vi "WILT.vi"() -> ()   [LabVIEW 2016] (continued)
                n1233 = Not(x=w2304) -> (.not. x?=w2315:bool)
                n1234 = call "WILT Agilent Valve Control.vi"("Station In"=w2316, "Agilent Channels In"=w2312, "Semaphore"=w2314, "Search"=T19 "Start Button", "Open/Close (F:Close)"=w2315, "error in (no error)"=w2311, "Test Type"=w2307, "Number Of Cycles"=w2306, "Cycle Time (mS)"=w2305) -> ("error out"=w2310:errorcluster)  [unwired: 4 in, 2 out]
              }
            }
            n1235 = call <vilib>:"Add State(s) to Queue__jki_lib_state_machine.vi"("State(s) in (\"\")"=w2302) -> ("States Out"=w2301:string)  [unwired: 14 in]
          }
          event Value Change {
            n1236 = event-data() -> ("NewVal"=w2317:bool)  [unwired: 1 in, 1 out]
            n1237 = case shown="False" w2317 {
              tunnel: w2320 -> [_ w2333]
              tunnel: w2319 -> [w2323 w2331]
              tunnel: [w2323 w2330] -> w2318
              tunnel: w2317 -> [_ w2324]
              frame False {
              }
              frame True {
                n1238 = local read "Number of ON/OFF Cycles"() -> (w2326:i32)
                n1239 = local read "Valve ON Time (mS)"() -> (w2325:u32)
                n1240 = local read "Agilent Semaphore"() -> (w2334:T1[])
                n1241 = Unbundle By Name(w2333) -> ("Agilent Switches"=w2332:T2[])
                n1242 = local read "Test Type"() -> (w2327:T12)
                n1243 = Number To Decimal String(number=55) -> (decimal integer string=w2336:string)  [unwired: 1 in]
                n1244 = Not(x=w2324) -> (.not. x?=w2335:bool)
                n1245 = call "WILT Agilent Valve Control.vi"("Station In"=w2336, "Agilent Channels In"=w2332, "Semaphore"=w2334, "Search"=T19 "Start Button", "Open/Close (F:Close)"=w2335, "error in (no error)"=w2331, "Test Type"=w2327, "Number Of Cycles"=w2326, "Cycle Time (mS)"=w2325) -> ("error out"=w2330:errorcluster)  [unwired: 4 in, 2 out]
              }
            }
            n1246 = call <vilib>:"Add State(s) to Queue__jki_lib_state_machine.vi"("State(s) in (\"\")"=w2322) -> ("States Out"=w2321:string)  [unwired: 14 in]
          }
          event Value Change {
            n1247 = event-data() -> ("NewVal"=w2337:bool)  [unwired: 1 in, 1 out]
            n1248 = case shown="False" w2337 {
              tunnel: w2340 -> [_ w2353]
              tunnel: w2339 -> [w2343 w2351]
              tunnel: [w2343 w2350] -> w2338
              tunnel: w2337 -> [_ w2344]
              frame False {
              }
              frame True {
                n1249 = local read "Number of ON/OFF Cycles"() -> (w2346:i32)
                n1250 = local read "Valve ON Time (mS)"() -> (w2345:u32)
                n1251 = local read "Agilent Semaphore"() -> (w2354:T1[])
                n1252 = Unbundle By Name(w2353) -> ("Agilent Switches"=w2352:T2[])
                n1253 = local read "Test Type"() -> (w2347:T12)
                n1254 = Number To Decimal String(number=56) -> (decimal integer string=w2356:string)  [unwired: 1 in]
                n1255 = Not(x=w2344) -> (.not. x?=w2355:bool)
                n1256 = call "WILT Agilent Valve Control.vi"("Station In"=w2356, "Agilent Channels In"=w2352, "Semaphore"=w2354, "Search"=T19 "Start Button", "Open/Close (F:Close)"=w2355, "error in (no error)"=w2351, "Test Type"=w2347, "Number Of Cycles"=w2346, "Cycle Time (mS)"=w2345) -> ("error out"=w2350:errorcluster)  [unwired: 4 in, 2 out]
              }
            }
            n1257 = call <vilib>:"Add State(s) to Queue__jki_lib_state_machine.vi"("State(s) in (\"\")"=w2342) -> ("States Out"=w2341:string)  [unwired: 14 in]
          }
          event User Event {
            n1258 = event-data() -> ()  [unwired: 1 in, 3 out]
            n1259 = Unbundle By Name(w2362) -> ("GUI Aisle 1 (SLAT)."=w2359:T3[])
            n1260 = local read "Aisle 1 Update"() -> (w2357:T3)
            n1261 = local read "Aisle 1 Location"() -> (w2358:i32)
            n1262 = call "WILT Update Aisle Info.vi"("Aisle 4 Update"=w2357, "Aisle 4 Location"=w2358, "GUI Aisle 4. in"=w2359) -> ("GUI Aisle 4. out"=w2360:T3[])  [unwired: 8 in]
            n1263 = Bundle By Name(cluster=w2362, "GUI Aisle 1 (SLAT)."=w2360) -> (w2361:T24)
          }
          event User Event {
            n1264 = event-data() -> ()  [unwired: 1 in, 5 out]
            n1265 = Unbundle By Name(w2370) -> ("GUI Aisle 1A (SLAT)."=w2367:T3[])
            n1266 = local read "Aisle 1A Location"() -> (w2366:i32)
            n1267 = local read "Aisle 1A Update"() -> (w2365:T3)
            n1268 = call "WILT Update Aisle Info.vi"("Aisle 4 Update"=w2365, "Aisle 4 Location"=w2366, "GUI Aisle 4. in"=w2367) -> ("GUI Aisle 4. out"=w2368:T3[])  [unwired: 8 in]
            n1269 = Bundle By Name(cluster=w2370, "GUI Aisle 1A (SLAT)."=w2368) -> (w2369:T24)
          }
          event User Event {
            n1270 = event-data() -> ()  [unwired: 1 in, 5 out]
            n1271 = Unbundle By Name(w2378) -> ("GUI Aisle 2."=w2375:T3[])
            n1272 = local read "Aisle 2 Location"() -> (w2374:i32)
            n1273 = local read "Aisle 2 Update"() -> (w2373:T3)
            n1274 = call "WILT Update Aisle Info.vi"("Aisle 4 Update"=w2373, "Aisle 4 Location"=w2374, "GUI Aisle 4. in"=w2375) -> ("GUI Aisle 4. out"=w2376:T3[])  [unwired: 8 in]
            n1275 = Bundle By Name(cluster=w2378, "GUI Aisle 2."=w2376) -> (w2377:T24)
          }
          event User Event {
            n1276 = event-data() -> ()  [unwired: 1 in, 5 out]
            n1277 = Unbundle By Name(w2386) -> ("GUI Aisle 3."=w2383:T3[])
            n1278 = local read "Aisle 3 Location"() -> (w2382:i32)
            n1279 = local read "Aisle 3 Update"() -> (w2381:T3)
            n1280 = call "WILT Update Aisle Info.vi"("Aisle 4 Update"=w2381, "Aisle 4 Location"=w2382, "GUI Aisle 4. in"=w2383) -> ("GUI Aisle 4. out"=w2384:T3[])  [unwired: 8 in]
            n1281 = Bundle By Name(cluster=w2386, "GUI Aisle 3."=w2384) -> (w2385:T24)
          }
          event User Event {
            n1282 = event-data() -> ()  [unwired: 1 in, 5 out]
            n1283 = local read "Aisle 4 Location"() -> (w2389:i32)
            n1284 = local read "Aisle 4 Update"() -> (w2391:T3)
            n1285 = Unbundle By Name(w2394) -> ("GUI Aisle 4."=w2390:T3[])
            n1286 = call "WILT Update Aisle Info.vi"("Aisle 4 Update"=w2391, "Aisle 4 Location"=w2389, "GUI Aisle 4. in"=w2390) -> ("GUI Aisle 4. out"=w2392:T3[])  [unwired: 8 in]
            n1287 = Bundle By Name(cluster=w2394, "GUI Aisle 4."=w2392) -> (w2393:T24)
          }
          event Value Change {
            n1288 = event-data() -> ("NewVal"=w2398:T11)  [unwired: 1 in, 5 out]
            n1289 = case shown="\"Night Cycle\"" w2398 {
              tunnel: ["Reset Start Retry" ("State(s) in Front (\"\")") "Reset Start Retry\nShutdown All Valves" ("State(s) in Front (\"\")")] -> w2397
              frame "Day Cycle", Default {
              }
              frame "Night Cycle" {
              }
            }
            n1290 = call <vilib>:"Add State(s) to Queue__jki_lib_state_machine.vi"("State(s) in Front (\"\")"=w2397, "State(s) in (\"\")"=w2400) -> ("States Out"=w2399:string)  [unwired: 13 in]
          }
          event "Shutdown All Valves": Value Change {
            n1291 = event-data() -> ("NewVal"=w2406:bool)  [unwired: 1 in, 5 out]
            n1292 = case shown="True" w2406 {
              tunnel: ["" ("State(s) in Front (\"\")") "Shutdown All Valves" ("State(s) in Front (\"\")")] -> w2405
              frame False {
              }
              frame True {
                n1293 = local write "Shutdown All Valves"(FALSE ("Shutdown All Valves")) -> ()
              }
            }
            n1294 = call <vilib>:"Add State(s) to Queue__jki_lib_state_machine.vi"("State(s) in Front (\"\")"=w2405, "State(s) in (\"\")"=w2408) -> ("States Out"=w2407:string)  [unwired: 13 in]
          }
          event "Reset Start Retry": Value Change {
            n1295 = event-data() -> ("NewVal"=w2415:bool)  [unwired: 1 in, 5 out]
            n1296 = case shown="True" w2415 {
              tunnel: ["" ("State(s) in Front (\"\")") "Reset Start Retry" ("State(s) in Front (\"\")")] -> w2414
              frame False {
              }
              frame True {
                n1297 = local write "Reset Start Retry"(FALSE ("Reset Start Retry")) -> ()
              }
            }
            n1298 = call <vilib>:"Add State(s) to Queue__jki_lib_state_machine.vi"("State(s) in Front (\"\")"=w2414, "State(s) in (\"\")"=w2417) -> ("States Out"=w2418:string)  [unwired: 13 in]
          }
          event "Reset Start Retry All True": Value Change {
            n1299 = event-data() -> ("NewVal"=w2424:bool)  [unwired: 1 in, 5 out]
            n1300 = case shown="True" w2424 {
              tunnel: ["" ("State(s) in Front (\"\")") "Reset Restart All True" ("State(s) in Front (\"\")")] -> w2423
              frame False {
              }
              frame True {
                n1301 = local write "Reset Start Retry All True"(FALSE ("Reset Start Retry")) -> ()
              }
            }
            n1302 = call <vilib>:"Add State(s) to Queue__jki_lib_state_machine.vi"("State(s) in Front (\"\")"=w2423, "State(s) in (\"\")"=w2426) -> ("States Out"=w2427:string)  [unwired: 13 in]
          }
          event "ExitProg": Value Change {
            n1303 = event-data() -> ()  [unwired: 1 in, 1 out]
            n1304 = call <vilib>:"Add State(s) to Queue__jki_lib_state_machine.vi"("State(s) in Front (\"\")"="Shutdown All Valves\nMacro: Exit", "State(s) in (\"\")"=w2436) -> ("States Out"=w2435:string)  [unwired: 13 in]
          }
          event Panel Close? {
            # "Discard the event because we'll close the front panel ourselves in Macro: Exit"
            # "Close Panel button (pressed) Event\n(this executes Macro: Exit to terminate the VI)"
            n1305 = event-data() -> ()  [unwired: 1 in, 1 out]
            n1306 = event-data("Discard?"=TRUE) -> ()  [unwired: 1 in, 1 out]
            n1307 = call <vilib>:"Add State(s) to Queue__jki_lib_state_machine.vi"("State(s) in Front (\"\")"="Macro: Exit", "State(s) in (\"\")"=w2442) -> ("States Out"=w2441:string)  [unwired: 13 in]
          }
        }
      }
      frame "---------- Core ----------" {
        n1308 = call <vilib>:"Add State(s) to Queue__jki_lib_state_machine.vi"("State(s) in (\"\")"=w2447) -> ("States Out"=w2446:string)  [unwired: 14 in]
      }
      frame Default {
        w2458 = 42 items=["No error", "Argument error", "Memory is full", "Out of zone", "End of file", "File already open", "Generic file I/O error", "File not found", "File permission error", "Disk is full", "Duplicate path", "Too many files open", "System feature not enabled", "Resource file not found", "Cannot add resource", "Resource not found", "Image not found", "Image memory error", "Pen does not exist", "Config type invalid", "Config token not found", "Config parse error", "Config memory error", "Bad external code format", "Bad external code offset", "External code not present", "Null window", "Destroy window error", "Null menu", "Print aborted", "Bad print record", "Print driver error", "Windows error during printing", "Memory error during printing", "Print dialog error", "Generic print error", "Invalid device refnum", "Device not found", "Device parameter error", "Device unit error", "Cannot open device", "Device call aborted", "Generic error", "Cancelled by user", "Object ID too low", "Object ID too high", "Object not in heap", "Unknown heap", "Unknown object (invalid DefProc)", "Unknown object (DefProc not in table)", "Message out of range", "Invalid (null) method", "Unknown message", "Manager call not supported", "Bad address", "Network operation in progress", "Network operation timed out", "Connection is busy", "Network attribute not supported", "Network error", "Address in use", "System out of memory", "Connection aborted", "Connection refused", "Not connected", "Already connected", "Connection closed", "Initialization error (interapplication manager)", "Bad occurrence", "Wait on unbound occurrence handler", "Occurrence queue overflow", "Datalog type conflict", "Unused", "Unrecognized type (interapplication manager)", "Memory corrupt", "Failed to make temporary DLL", "Old CIN version", "Drag socket not found", "Failed to load drop-object", "Failed to register OLE object", "Failed to release OLE object", "Format specifier type mismatch", "Unknown format specifier", "Too few format specifiers", "Too many format specifiers", "Scan failed", "Newer CIN version", "Error converting to variant", "Runtime menu error", "Password tampered", "Variant attribute not found", "Incompatible variant data type", "Event data is not available", "Event Store is not present", "Occurrence is not found", "Event Queue is not created", "Event info is not available", "Refnum passed is NULL", "Error retrieving Class GUID", "Error retrieving CoClass GUID", "Error retrieving TypeLib GUID.", "Bad built application magic bytes.", "Specific driver is different from the specific driver associated with the Logical Name.", "There is no session opened to the class driver.", "Max Error", "MAX - Error with config objects", "MAX - Error loading configuration", "MAX - Group not supported"]
        # "Current State"
        # "Do not delete, rename, or modify this frame.\n(this is used to capture unhandled states and typos)"
        # "Handle mistyped state name (developer tool)"
        n1309 = Format Into String(format string="Software Exception: Unhandled State \"%s\"." ("message"), error in=w2454, w2449) -> (resulting string=w2457:string, error out=w2456:errorcluster)  [unwired: 1 in]
        n1310 = call <vilib>:"Error Cluster From Error Code.vi"("show call chain? (False)"=TRUE, "error in (no error)"=w2456, "error message (\"\")"=w2457, "error code (0)"=w2458) -> ("error out"=w2455:errorcluster)  [unwired: 5 in]
        n1311 = call <vilib>:"Add State(s) to Queue__jki_lib_state_machine.vi"("State(s) in (\"\")"=w2453) -> ("States Out"=w2452:string)  [unwired: 14 in]
      }
      frame "Initialize Core Data" {
        # "Do not delete, rename, or modify this frame.\n(this is used to determine panel behavior on exit)"
        # "originally closed?"
        # "exe?"
        # "If panel starts closed or is an EXE, then close it when we exit"
        n1312 = property class="VI"() -> ("Front Panel.Open"=w2468:bool)  [unwired: 2 in, 2 out]
        n1313 = property class="App"() -> ("App.Kind"=w2467:T20)  [unwired: 2 in, 2 out]
        n1314 = control-ref of="Current VI Reference"() -> (w2461:refnum<vi>)
        n1315 = Not(x=w2468) -> (.not. x?=w2465:bool)
        n1316 = Equal?(x=w2467, y=T20."Run Time System" ("Application:Kind")) -> (x = y?=w2464:bool)
        n1317 = Or(x=w2465, y=w2464) -> (x .or. y?=w2462:bool)
        n1318 = Bundle By Name(cluster=w2463, "Core.Current VI Reference"=w2461, "Core.Close Panel on Exit?"=w2462) -> (w2470:T24)
        n1319 = call <vilib>:"Add State(s) to Queue__jki_lib_state_machine.vi"("State(s) in (\"\")"=w2472) -> ("States Out"=w2471:string)  [unwired: 14 in]
      }
      frame "Error Handler" {
        # "Unhandled Error -- Display it"
        # "Handle any errors here.\nYou can also output any states to clean-up after errors occur"
        # "Clear error"
        n1320 = call <vilib>:"General Error Handler.vi"("error in (no error)"=w2475) -> ()  [unwired: 10 in, 5 out]
        n1321 = call <vilib>:"Add State(s) to Queue__jki_lib_state_machine.vi"("State(s) in Front (\"\")"="/* Post Error States", "State(s) in (\"\")"=w2479) -> ("States Out"=w2478:string)  [unwired: 13 in]
      }
      frame "Exit" {
        # "Do not put any code in this frame.\n(No errors that occur here will be handled.)"
        n1322 = call <vilib>:"Add State(s) to Queue__jki_lib_state_machine.vi"("State(s) in (\"\")"=w2485) -> ("States Out"=w2484:string)  [unwired: 14 in]
      }
      frame "---------- Data ----------" {
        # "Do not put any code in this frame.\n(It is a separator no-op. You can make a copy of this frame to create a new Data frame)"
        n1323 = call <vilib>:"Add State(s) to Queue__jki_lib_state_machine.vi"("State(s) in (\"\")"=w2490) -> ("States Out"=w2489:string)  [unwired: 14 in]
      }
      frame "Data: Initialize" {
        w2495 = 0.0  # Send Restart Every? (Sec)
        w2496 = bool[] [FALSE, FALSE, FALSE, FALSE, FALSE, FALSE, FALSE, FALSE, FALSE, FALSE, FALSE, FALSE, FALSE, FALSE, FALSE, FALSE, FALSE, FALSE, FALSE, FALSE, FALSE, FALSE, FALSE, FALSE, FALSE, FALSE, FALSE, FALSE, FALSE, FALSE, FALSE, FALSE, FALSE, FALSE, FALSE, FALSE, FALSE, FALSE, FALSE, FALSE, FALSE, FALSE, FALSE, FALSE, FALSE, FALSE, FALSE, FALSE, FALSE, FALSE, FALSE, FALSE, FALSE, FALSE, FALSE, FALSE]  # Enable Start Retry Array
        w2500 = 1.0  # Current Threshold
        w2512 = T25 {"Current VI Reference"=refnum, "Close Panel on Exit?"=FALSE}  # Core
        n1324 = Bundle("Send Restart Every? (Sec)"=w2495, "Enable Start Retry Array"=w2496, "Agilent Switches"="Agilent Switches", "States"="", "Core"=w2512, "Station Test State Cluster"="Station Test State Cluster", "GUI Aisle 4."="GUI Aisle 4.", "GUI Aisle 3."="GUI Aisle 3.", "GUI Aisle 2."="GUI Aisle 2.", "GUI Aisle 1A (SLAT)."="GUI Aisle 1A (SLAT).", "GUI Aisle 1 (SLAT)."="GUI Aisle 1 (SLAT).", "Agilent Refs"="Agilent Refs", "Configuration Startup Directorys"=T21 {"Debug File DIR"="", "Inverter And MC File DIR"=""}, "File Locations"="File Locations", "Day/Night Cycle Input"=WILT_Day_Night_Cycle_Enum."Day Cycle", "Injection Times Input"=T15 [], "Current Threshold"=w2500, "Station Timeout Values (1-56) Seconds"="Station Timeout Values (1-56) Seconds", "Drying Time (Min)"="Drying Time (Min)") -> (w2492:T24)  [unwired: 1 in]
        n1325 = call <vilib>:"Add State(s) to Queue__jki_lib_state_machine.vi"("State(s) in (\"\")"=w2514) -> ("States Out"=w2513:string)  [unwired: 14 in]
      }
      frame "Data: Cleanup" {
        # "Cleanup any data and references, here.\n(this is called automatically, by the Macro: Exit)"
        n1326 = Unbundle By Name(w2516) -> ("Core.Current VI Reference"=w2519:refnum<vi>)
        n1327 = Close Reference(reference=w2519, error in (no error)=w2518) -> (error out=w2517:errorcluster)
        n1328 = call <vilib>:"Add State(s) to Queue__jki_lib_state_machine.vi"("State(s) in (\"\")"=w2521) -> ("States Out"=w2520:string)  [unwired: 14 in]
      }
      frame "---------- UI ----------" {
        # "Do not put any code in this frame.\n(It is a separator no-op. You can make a copy of this frame to create a new UI frame)"
        n1329 = call <vilib>:"Add State(s) to Queue__jki_lib_state_machine.vi"("State(s) in (\"\")"=w2526) -> ("States Out"=w2525:string)  [unwired: 14 in]
      }
      frame "UI: Initialize" {
        # "Initialize everything so it starts without a serial number.\nThis prevents from running"
        n1330 = Current VI's Path() -> (path=w2531:path)
        n1331 = Unbundle By Name(w2533) -> ("File Locations"=w2532:T17[])
        n1332 = call "UTILITY This VIs Path.vi"("path"=w2531, "error in (no error)"=w2530) -> ("Folder Path"=w2528:path, "error out"=w2529:errorcluster)  [unwired: 7 in, 5 out]
        n1333 = for {
          tunnel: w2532 -> [w2547] mode=indexing
          tunnel: w2528 -> [w2546]
          tunnel: [w2545] -> w2527 mode=indexing
          n1334 = Bundle By Name(cluster=w2547, "General Setup Paths.Tool Base Path"=w2546) -> (w2545:T17)
        }
        n1335 = Initialize Array(T3 {"Lab ID"="", "Day Cycle Count"=0, "Station Label"="", "Dryer Details"={"Station"="", "Lab ID"="", "TR Number"=""}, "Status Color"=0, "Invisible Button"=FALSE, "Night Cycle Count"=0, "Station Index"=0, "Cycle Index"="", "Audit Alert"=FALSE, "Agilent Channel Definition"={"Channel"="", "Station"="", "Label"="", "Agilent Station"="", "Data"=0.0}, "DAQ Data"={"L1 Current"=0.0, "L2 Current"=0.0, "Temperature  Deg F (TC)"=0.0, "Volts"=0.0, "Volts (208)"=0.0, "SW (208)"=0.0}} ("Initial Dryer Cluster"), 12 ("dimension size")) -> (w2539:T3[])
        n1336 = Initialize Array(T3 {"Lab ID"="", "Day Cycle Count"=0, "Station Label"="", "Dryer Details"={"Station"="", "Lab ID"="", "TR Number"=""}, "Status Color"=0, "Invisible Button"=FALSE, "Night Cycle Count"=0, "Station Index"=0, "Cycle Index"="", "Audit Alert"=FALSE, "Agilent Channel Definition"={"Channel"="", "Station"="", "Label"="", "Agilent Station"="", "Data"=0.0}, "DAQ Data"={"L1 Current"=0.0, "L2 Current"=0.0, "Temperature  Deg F (TC)"=0.0, "Volts"=0.0, "Volts (208)"=0.0, "SW (208)"=0.0}} ("Initial Dryer Cluster"), 8 ("dimension size")) -> (w2536:T3[])
        n1337 = Bundle By Name(cluster=w2533, "Station Test State Cluster"=T7 {"Station Test State 1"=enum."No Serial Number", "Station Test State 2"=enum."No Serial Number", "Station Test State 3"=enum."No Serial Number", "Station Test State 4"=enum."No Serial Number", "Station Test State 5"=enum."No Serial Number", "Station Test State 6"=enum."No Serial Number", "Station Test State 7"=enum."No Serial Number", "Station Test State 8"=enum."No Serial Number", "Station Test State 9"=enum."No Serial Number", "Station Test State 10"=enum."No Serial Number", "Station Test State 11"=enum."No Serial Number", "Station Test State 12"=enum."No Serial Number", "Station Test State 13"=enum."No Serial Number", "Station Test State 14"=enum."No Serial Number", "Station Test State 15"=enum."No Serial Number", "Station Test State 16"=enum."No Serial Number", "Station Test State 17"=enum."No Serial Number", "Station Test State 18"=enum."No Serial Number", "Station Test State 19"=enum."No Serial Number", "Station Test State 20"=enum."No Serial Number", "Station Test State 21"=enum."No Serial Number", "Station Test State 22"=enum."No Serial Number", "Station Test State 23"=enum."No Serial Number", "Station Test State 24"=enum."No Serial Number", "Station Test State 25"=enum."No Serial Number", "Station Test State 26"=enum."No Serial Number", "Station Test State 27"=enum."No Serial Number", "Station Test State 28"=enum."No Serial Number", "Station Test State 29"=enum."No Serial Number", "Station Test State 30"=enum."No Serial Number", "Station Test State 31"=enum."No Serial Number", "Station Test State 32"=enum."No Serial Number", "Station Test State 33"=enum."No Serial Number", "Station Test State 34"=enum."No Serial Number", "Station Test State 35"=enum."No Serial Number", "Station Test State 36"=enum."No Serial Number", "Station Test State 37"=enum."No Serial Number", "Station Test State 38"=enum."No Serial Number", "Station Test State 39"=enum."No Serial Number", "Station Test State 40"=enum."No Serial Number", "Station Test State 41"=enum."No Serial Number", "Station Test State 42"=enum."No Serial Number", "Station Test State 43"=enum."No Serial Number", "Station Test State 44"=enum."No Serial Number", "Station Test State 45"=enum."No Serial Number", "Station Test State 46"=enum."No Serial Number", "Station Test State 47"=enum."No Serial Number", "Station Test State 48"=enum."No Serial Number", "Station Test State 49"=enum."No Serial Number", "Station Test State 50"=enum."No Serial Number", "Station Test State 51"=enum."No Serial Number", "Station Test State 52"=enum."No Serial Number", "Station Test State 53"=enum."No Serial Number", "Station Test State 54"=enum."No Serial Number", "Station Test State 55"=enum."No Serial Number", "Station Test State 56"=enum."No Serial Number"}, "GUI Aisle 4."=w2539, "GUI Aisle 3."=w2539, "GUI Aisle 2."=w2539, "GUI Aisle 1 (SLAT)."=w2539, "GUI Aisle 1A (SLAT)."=w2536, "File Locations"=w2527) -> (w2542:T24)
        n1338 = call <vilib>:"Add State(s) to Queue__jki_lib_state_machine.vi"("State(s) in (\"\")"=w2544) -> ("States Out"=w2543:string)  [unwired: 14 in]
      }
      frame "Read General Config" {
        # "Populate the general file path settings"
        n1339 = Unbundle By Name(w2555) -> ("File Locations"=w2550:T17[])
        n1340 = call "WILT Read General Configuration.vi"("File Path Input"=w2550, "Error In"=w2559) -> ("Scan Rate"=w2554:dbl, "Save Rate"=w2553:dbl, "Current Threshold"=w2552:dbl, "Send Restart Every? (Sec)"=w2551:dbl, "State Machine String"=w2557:string, "File Path Output"=w2549:T17[], "Station Timeout Values (1-56) Seconds"=w2556:dbl[], "Drying Time (Min)"=w2548:dbl[], "Error Out"=w2558:errorcluster)  [unwired: 9 in]
        n1341 = local write "Drying Time (Min)"(w2548) -> ()
        n1342 = Bundle By Name(cluster=w2555, "Send Restart Every? (Sec)"=w2551, "States"=w2557, "File Locations"=w2549, "Station Timeout Values (1-56) Seconds"=w2556, "Drying Time (Min)"=w2548) -> (w2561:T24)
        n1343 = local write "Scan Rate (Seconds)"(w2554) -> ()
        n1344 = local write "Save Rate (Seconds)"(w2553) -> ()
        n1345 = local write "Current Threshold"(w2552) -> ()
        n1346 = call <vilib>:"Add State(s) to Queue__jki_lib_state_machine.vi"("State(s) in (\"\")"=w2563) -> ("States Out"=w2562:string)  [unwired: 14 in]
      }
      frame "Read Previous" {
        n1347 = Unbundle By Name(w2571) -> ("File Locations"=w2564:T17[], "GUI Aisle 4."=w2566:T3[], "GUI Aisle 3."=w2567:T3[], "GUI Aisle 2."=w2568:T3[], "GUI Aisle 1 (SLAT)."=w2569:T3[], "GUI Aisle 1A (SLAT)."=w2570:T3[])
        n1348 = call "WILT Stave Status.vi"("GUI Aisle 4"=w2566, "Operation Type"=enum16{"Write", "Read"}."Read", "File Locations"=w2564, "GUI Aisle 3"=w2567, "GUI Aisle 2"=w2568, "GUI Aisle 1 (SLAT)"=w2569, "Error In"=w2578, "GUI Aisle 1A (SLAT)"=w2570) -> ("GUI Aisle 4 Out"=w2576:T3[], "GUI Aisle 3 Out"=w2575:T3[], "GUI Aisle 2 Out"=w2574:T3[], "GUI Aisle 1 (SLAT) Out"=w2573:T3[], "GUI Aisle 1A (SLAT) Out"=w2572:T3[], "Error Out"=w2577:errorcluster)  [unwired: 2 in]
        n1349 = local write "GUI Aisle 4."(w2576) -> ()
        n1350 = local write "GUI Aisle 3."(w2575) -> ()
        n1351 = local write "GUI Aisle 2."(w2574) -> ()
        n1352 = local write "GUI Aisle 1 (SLAT)."(w2573) -> ()
        n1353 = local write "GUI Aisle 1A (SLAT)."(w2572) -> ()
        n1354 = Bundle By Name(cluster=w2571, "GUI Aisle 4."=w2576, "GUI Aisle 3."=w2575, "GUI Aisle 2."=w2574, "GUI Aisle 1 (SLAT)."=w2573, "GUI Aisle 1A (SLAT)."=w2572) -> (w2580:T24)
        n1355 = call <vilib>:"Add State(s) to Queue__jki_lib_state_machine.vi"("State(s) in (\"\")"=w2582) -> ("States Out"=w2581:string)  [unwired: 14 in]
      }
      frame "Read Water Times" {
        n1356 = Unbundle By Name(w2586) -> ("File Locations"=w2587:T17[])
        n1357 = call "WILT Watering Times.vi"("Execution Type"=enum16{"Write", "Read"}."Read", "File Locations"=w2587) -> ("Watering Times Output"=w2585:T15)  [unwired: 8 in, 1 out]
        n1358 = local write "Injection Times"(w2585) -> ()
        n1359 = call <vilib>:"Add State(s) to Queue__jki_lib_state_machine.vi"("State(s) in (\"\")"=w2590) -> ("States Out"=w2589:string)  [unwired: 14 in]
      }
      frame "UI: Cursor Set" {
        # "Argument"
        n1360 = case shown="\"Idle\", Default" w2592 {
          tunnel: w2594 -> [w2599 w2601]
          tunnel: [w2598 w2600] -> w2593
          frame "Idle", Default {
            n1361 = call <vilib>:"Unset Busy.vi"("error in (no error)"=w2599) -> ("error out"=w2598:errorcluster)  [unwired: 10 in]
          }
          frame "Busy" {
            n1362 = call <vilib>:"Set Busy.vi"("error in (no error)"=w2601) -> ("error out"=w2600:errorcluster)  [unwired: 9 in, 1 out]
          }
        }
        n1363 = call <vilib>:"Add State(s) to Queue__jki_lib_state_machine.vi"("State(s) in (\"\")"=w2597) -> ("States Out"=w2596:string)  [unwired: 14 in]
      }
      frame "UI: Front Panel State" {
        # "Argument"
        # "Set Front Panel Open or Closed\n(Usage: \"UI: Front Panel State >> Open|Close\")"
        n1364 = Unbundle By Name(w2605) -> ("Core.Current VI Reference"=w2604:refnum<vi>)
        n1365 = case shown="\"Open\", Default" w2603 {
          tunnel: w2607 -> [w2613 w2626]
          tunnel: [w2615 w2627] -> w2606
          tunnel: w2604 -> [w2614 w2624]
          frame "Open", Default {
            n1366 = property class="VI"(reference=w2614, error in=w2613) -> (reference out=w2611:refnum<vi>, error out=w2612:errorcluster, "Front Panel.Open"=w2610:bool)
            n1367 = case shown="False" w2610 {
              tunnel: [w2618 w2621] -> w2615
              tunnel: w2612 -> [w2617 w2621]
              tunnel: w2611 -> [w2616 _]
              frame False {
                n1368 = invoke class="VI" method="FP.Open"(reference=w2616, error in=w2617, "Activate"=TRUE, "State"=T22."Standard") -> (error out=w2618:errorcluster)  [unwired: 1 in, 4 out]
              }
              frame True {
              }
            }
          }
          frame "Close" {
            n1369 = property class="VI"(reference=w2624, error in=w2626) -> (reference out=w2623:refnum<vi>, error out=w2625:errorcluster, "Front Panel.Open"=w2622:bool)
            n1370 = case shown="True" w2622 {
              tunnel: [w2628 w2631] -> w2627
              tunnel: w2625 -> [w2628 w2630]
              tunnel: w2623 -> [_ w2629]
              frame False {
              }
              frame True {
                n1371 = invoke class="VI" method="FP.Close"(reference=w2629, error in=w2630) -> (error out=w2631:errorcluster)  [unwired: 1 in, 2 out]
              }
            }
          }
        }
        n1372 = call <vilib>:"Add State(s) to Queue__jki_lib_state_machine.vi"("State(s) in (\"\")"=w2609) -> ("States Out"=w2608:string)  [unwired: 14 in]
      }
      frame "Initialize Agilents" {
        n1373 = local read "Agilent Semaphore"() -> (w2634:T1[])
        n1374 = Unbundle By Name(w2637) -> ("File Locations"=w2633:T17[], "Agilent Refs"=w2642:refnum<visa-resource-name>[])
        n1375 = call "WILT Agilent Setup.vi"("Custom Agilent List"=FALSE, "Agilent Semaphore"=w2634, "error in (no error)"=w2641, "Agilent Refs"=w2642, "File Locations"=w2633) -> ("error out"=w2640:errorcluster, "Data Out Array"=→"Data Out Array":T6, "Agilent Switches"=w2635:T2[])  [unwired: 4 in]
        n1376 = Bundle By Name(cluster=w2637, "Agilent Switches"=w2635) -> (w2636:T24)
        n1377 = call <vilib>:"Add State(s) to Queue__jki_lib_state_machine.vi"("State(s) in (\"\")"=w2644) -> ("States Out"=w2643:string)  [unwired: 14 in]
      }
      frame "Initialize File Names" {
        # "Dont create folders if Lab ID is blank"
        n1378 = Unbundle By Name(w2645) -> ("File Locations"=w2646:T17[], "GUI Aisle 1 (SLAT)."=w2658:T3[], "GUI Aisle 1A (SLAT)."=w2657:T3[], "GUI Aisle 2."=w2656:T3[], "GUI Aisle 3."=w2655:T3[], "GUI Aisle 4."=w2654:T3[])
        n1379 = Build Array (concatenate)(w2658, w2657, w2656, w2655, w2654) -> (w2653:T3[])
        n1380 = for {
          tunnel: w2653 -> [w2668] mode=indexing
          tunnel: [w2667] -> w2651 mode=indexing
          tunnel: w2646 -> [w2662] mode=indexing
          n1381 = call "WILT Dryer To Washer Control Converter File Save.vi"("Dryer 14"=w2668) -> ("Initialize.Washer In"=w2663:T26)  [unwired: 9 in, 1 out]
          n1382 = Unbundle By Name(w2663) -> ("Appliance Details.Appliance Common.Lab ID:"=w2664:string)
          n1383 = Equal?(x=w2664, y="") -> (x = y?=w2665:bool)
          n1384 = case shown="False" w2665 {
            tunnel: w2662 -> [w2672 w2673]
            tunnel: w2663 -> [w2671 _]
            tunnel: [w2670 w2673] -> w2667
            frame False {
              n1385 = call "Save File Create Filename and Directories.vi"("LV Program"=Save_File_DOE_LabView_Program."Dryer WILT", "Initialize.Washer In"=w2671, "File Paths In"=w2672) -> ("File Paths Out"=w2670:T17)  [unwired: 6 in, 2 out]
            }
            frame True {
            }
          }
        }
        n1386 = Initialize Array(refnum<file> refnum ("File Refnum"), 57 ("dimension size")) -> (→"File Refnums":refnum<file>[])
        n1387 = call <vilib>:"Add State(s) to Queue__jki_lib_state_machine.vi"("State(s) in (\"\")"=w2661) -> ("States Out"=w2660:string)  [unwired: 14 in]
        n1388 = Bundle By Name(cluster=w2645, "File Locations"=w2651) -> (w2652:T24)
        n1389 = local write "File Locations"(w2651) -> ()
      }
      frame "Shutdown All Valves" {
        n1390 = Unbundle By Name(w2683) -> ("Agilent Switches"=w2682:T2[])
        n1391 = global read "WILT Globals Main Program.vi" "Startup"() -> (→"Unused":u32)
        n1392 = global read "WILT Globals Main Program.vi" "Run"() -> (→"Running":u32)
        n1393 = global read "WILT Globals Main Program.vi" "Color Uncofigured"() -> (→"No Com":u32)
        n1394 = global read "WILT Globals Main Program.vi" "Problem"() -> (→"Fault":u32)
        n1395 = global read "WILT Globals Main Program.vi" "Pause"() -> (→"Stopped":u32)
        n1396 = global read "WILT Globals Main Program.vi" "Watering"() -> (→"Watering":u32)
        n1397 = global read "WILT Globals Main Program.vi" "EOC"() -> (→"Waiting For Start":u32)
        n1398 = local read "Agilent Semaphore"() -> (w2674:T1[])
        n1399 = call "WILT Shutdown All Valves.vi"("Agilent Semaphore"=w2674, "error in (no error)"=w2685, "Agilent Switches"=w2682) -> ("error out"=w2684:errorcluster)  [unwired: 8 in]
        n1400 = call <vilib>:"Add State(s) to Queue__jki_lib_state_machine.vi"("State(s) in (\"\")"=w2688) -> ("States Out"=w2687:string)  [unwired: 14 in]
      }
      frame "Initialization Complete" {
        n1401 = Current VI's Path() -> (path=w2695:path)
        n1402 = call "UTILITY This VIs Path.vi"("path"=w2695, "error in (no error)"=w2690) -> ("Robocopy Path"=w2691:string, "FileVersionInfo Out"=w2694:T28, "error out"=w2689:errorcluster)  [unwired: 7 in, 4 out]
        n1403 = Unbundle By Name(w2694) -> ("FileVersion"=→"Version":string)
        n1404 = call <vilib>:"System Exec.vi"("wait until completion? (T)"=FALSE, "command line"=w2691) -> ()  [unwired: 6 in, 4 out]
        n1405 = call <vilib>:"Add State(s) to Queue__jki_lib_state_machine.vi"("State(s) in (\"\")"=w2700) -> ("States Out"=w2699:string)  [unwired: 14 in]
        "Initialization Complete" <- TRUE ("Initialization Complete")
      }
      frame "Reset Start Retry" {
        n1406 = Initialize Array(FALSE, 56 ("dimension size")) -> (w2701:bool[])
        n1407 = Bundle By Name(cluster=w2705, "Enable Start Retry Array"=w2701) -> (w2704:T24)
        n1408 = call <vilib>:"Add State(s) to Queue__jki_lib_state_machine.vi"("State(s) in (\"\")"=w2709) -> ("States Out"=w2708:string)  [unwired: 14 in]
      }
      frame "Reset Restart All True" {
        n1409 = Initialize Array(TRUE, 56 ("dimension size")) -> (w2710:bool[])
        n1410 = Bundle By Name(cluster=w2714, "Enable Start Retry Array"=w2710) -> (w2713:T24)
        n1411 = call <vilib>:"Add State(s) to Queue__jki_lib_state_machine.vi"("State(s) in (\"\")"=w2718) -> ("States Out"=w2717:string)  [unwired: 14 in]
      }
      frame "Wait Seconds" {
        n1412 = call "UTILITY Delay mS.vi"("Error In"=w2721, "milliseconds to wait"=u32 20000) -> ("Error Out"=w2720:errorcluster)  [unwired: 13 in]
        n1413 = call <vilib>:"Add State(s) to Queue__jki_lib_state_machine.vi"("State(s) in (\"\")"=w2725) -> ("States Out"=w2724:string)  [unwired: 14 in]
      }
      frame "---------- Macro ----------" {
        # "Do not put any code in this frame.\n(It is a separator no-op. You can make a copy of this frame to create a new Macro frame)"
        n1414 = call <vilib>:"Add State(s) to Queue__jki_lib_state_machine.vi"("State(s) in (\"\")"=w2730) -> ("States Out"=w2729:string)  [unwired: 14 in]
      }
      frame "Macro: Initialize" {
        w2732 = "Data: Initialize\nInitialize Core Data\nUI: Initialize\nRead General Config\nRead Previous\nRead Water Times\nInitialize Agilents\nInitialize File Names\nShutdown All Valves\nInitialization Complete\nUI: Front Panel State >> Open"  # Data: Initialize Initialize Core Data UI: Initialize Read General Config Read Previous Read Water Times Initialize Agilents Initialize File Names Shutdown All Valves Initialization Complete UI: Front Panel State >> Open
        n1415 = call <vilib>:"Add State(s) to Queue__jki_lib_state_machine.vi"("State(s) in Front (\"\")"=w2732, "State(s) in (\"\")"=w2736) -> ("States Out"=w2735:string)  [unwired: 13 in]
      }
      frame "Macro: Exit" {
        # "Exit Macro\n(This is called once, when the VI exits)"
        n1416 = Unbundle By Name(w2744) -> ("Core.Close Panel on Exit?"=w2743:bool)
        n1417 = Select(t="UI: Front Panel State >> Close", s=w2743, f="") -> (s? t:f=w2740:string)
        n1418 = call <vilib>:"Add State(s) to Queue__jki_lib_state_machine.vi"("State(s) in (\"\")"=w2740, "State(s) at Back (\"\")"="Data: Cleanup\nExit") -> ("States Out"=w2738:string)  [unwired: 13 in]
        n1419 = call <vilib>:"Add State(s) to Queue__jki_lib_state_machine.vi"("State(s) in Front (\"\")"=w2738, "State(s) in (\"\")"=w2747) -> ("States Out"=w2746:string)  [unwired: 13 in]
      }
      frame "---------- New Category ----------" {
        # "Template Separator\n(You can make a copy of, or modify, this frame)"
        n1420 = call <vilib>:"Add State(s) to Queue__jki_lib_state_machine.vi"("State(s) in (\"\")"=w2752) -> ("States Out"=w2751:string)  [unwired: 14 in]
      }
      frame "Read Constants" {
        n1421 = Bundle By Name(cluster=w2757, "Day/Night Cycle Input"="Day/Night Cycle", "Injection Times Input"="Injection Times", "Current Threshold"="Current Threshold") -> (w2756:T24)
        n1422 = call <vilib>:"Add State(s) to Queue__jki_lib_state_machine.vi"("State(s) in (\"\")"=w2761) -> ("States Out"=w2760:string)  [unwired: 14 in]
      }
      frame "Station 1" {
        w2779 = 0  # Aisle Location Index
        w2782 = u32 1  # Station Number
        # "Clean this up with a control"
        # "Control the state of station 1"
        n1423 = Unbundle By Name(w2786) -> ("Enable Start Retry Array"=w2771:bool[], "Agilent Switches"=w2772:T2[], "GUI Aisle 1 (SLAT)."=w2784:T3[], "Drying Time (Min)"=w2766:dbl[], "Current Threshold"=w2773:dbl, "Station Test State Cluster"=w2777:T7, "Station Timeout Values (1-56) Seconds"=w2767:dbl[], "Send Restart Every? (Sec)"=w2769:dbl, "Injection Times Input"=w2774:T15, "Day/Night Cycle Input"=w2775:T11)
        n1424 = local read "Previous Run Statistics"() -> (w2768:T9[])
        n1425 = local read "Agilent Semaphore"() -> (w2765:T1[])
        n1426 = call "WILT Station Controller.vi"("Station Number"=w2782, "GUI Aisle in"=w2784, "Drying Time (Min)"=w2766, "Current Threshold"=w2773, "Station Test State In"=w2777, "Error In"=w2781, "Aisle Location Index"=w2779, "Cool Down Period (seconds)"=w2767, "Disable Flood Check"="Disable Flood Check", "Delay After Cutout (sec)"="Delay After Cutout (Sec)", "Previous Run Statistics"=w2768, "Send Restart Every? (Sec)"=w2769, "Agilent Valve and Switch Locations"=w2772, "Injection Times"=w2774, "Enable Start Retry"=w2771, "Day/Night Cycle"=w2775, "Final Start Presses"="Final Start Presses", "Semaphore"=w2765) -> ("GUI Aisle 1"=w2783:T3[], "Test Station Out"=w2778:T7, "Enable Start Retry Out"=w2770:bool[], "Error Out"=w2780:errorcluster)  [unwired: 5 in, 1 out]
        n1427 = Bundle By Name(cluster=w2786, "GUI Aisle 1 (SLAT)."=w2783, "Station Test State Cluster"=w2778, "Enable Start Retry Array"=w2770) -> (w2785:T24)
        n1428 = call <vilib>:"Add State(s) to Queue__jki_lib_state_machine.vi"("State(s) in (\"\")"=w2788) -> ("States Out"=w2787:string)  [unwired: 14 in]
      }
      frame "Station 2" {
        w2806 = 1  # Aisle Location Index
        w2809 = u32 2  # Station Number
        # "Control the state of station 2"
        n1429 = Unbundle By Name(w2813) -> ("Enable Start Retry Array"=w2797:bool[], "Agilent Switches"=w2799:T2[], "GUI Aisle 1 (SLAT)."=w2811:T3[], "Drying Time (Min)"=w2794:dbl[], "Current Threshold"=w2800:dbl, "Station Test State Cluster"=w2804:T7, "Station Timeout Values (1-56) Seconds"=w2795:dbl[], "Send Restart Every? (Sec)"=w2796:dbl, "Injection Times Input"=w2801:T15, "Day/Night Cycle Input"=w2802:T11)
        n1430 = local read "Disable Flood Check"() -> (w2789:bool)
        n1431 = local read "Delay After Cutout (Sec)"() -> (w2791:dbl)
        n1432 = local read "Final Start Presses"() -> (w2790:i32)
        n1433 = local read "Agilent Semaphore"() -> (w2792:T1[])
        n1434 = local read "Previous Run Statistics"() -> (w2793:T9[])
        n1435 = call "WILT Station Controller.vi"("Station Number"=w2809, "GUI Aisle in"=w2811, "Drying Time (Min)"=w2794, "Current Threshold"=w2800, "Station Test State In"=w2804, "Error In"=w2808, "Aisle Location Index"=w2806, "Cool Down Period (seconds)"=w2795, "Disable Flood Check"=w2789, "Delay After Cutout (sec)"=w2791, "Previous Run Statistics"=w2793, "Send Restart Every? (Sec)"=w2796, "Agilent Valve and Switch Locations"=w2799, "Injection Times"=w2801, "Enable Start Retry"=w2797, "Day/Night Cycle"=w2802, "Final Start Presses"=w2790, "Semaphore"=w2792) -> ("GUI Aisle 1"=w2810:T3[], "Test Station Out"=w2805:T7, "Enable Start Retry Out"=w2798:bool[], "Error Out"=w2807:errorcluster)  [unwired: 5 in, 1 out]
        n1436 = Bundle By Name(cluster=w2813, "GUI Aisle 1 (SLAT)."=w2810, "Station Test State Cluster"=w2805, "Enable Start Retry Array"=w2798) -> (w2812:T24)
        n1437 = call <vilib>:"Add State(s) to Queue__jki_lib_state_machine.vi"("State(s) in (\"\")"=w2815) -> ("States Out"=w2814:string)  [unwired: 14 in]
      }
      frame "Station 3" {
        w2833 = 2  # Aisle Location Index
        w2836 = u32 3  # Station Number
        # "Control the state of station 3"
        n1438 = Unbundle By Name(w2840) -> ("Enable Start Retry Array"=w2824:bool[], "Agilent Switches"=w2826:T2[], "GUI Aisle 1 (SLAT)."=w2838:T3[], "Drying Time (Min)"=w2820:dbl[], "Current Threshold"=w2827:dbl, "Station Test State Cluster"=w2831:T7, "Station Timeout Values (1-56) Seconds"=w2822:dbl[], "Send Restart Every? (Sec)"=w2823:dbl, "Injection Times Input"=w2828:T15, "Day/Night Cycle Input"=w2829:T11)
        n1439 = local read "Previous Run Statistics"() -> (w2821:T9[])
        n1440 = local read "Disable Flood Check"() -> (w2816:bool)
        n1441 = local read "Delay After Cutout (Sec)"() -> (w2818:dbl)
        n1442 = local read "Final Start Presses"() -> (w2817:i32)
        n1443 = local read "Agilent Semaphore"() -> (w2819:T1[])
        n1444 = call "WILT Station Controller.vi"("Station Number"=w2836, "GUI Aisle in"=w2838, "Drying Time (Min)"=w2820, "Current Threshold"=w2827, "Station Test State In"=w2831, "Error In"=w2835, "Aisle Location Index"=w2833, "Cool Down Period (seconds)"=w2822, "Disable Flood Check"=w2816, "Delay After Cutout (sec)"=w2818, "Previous Run Statistics"=w2821, "Send Restart Every? (Sec)"=w2823, "Agilent Valve and Switch Locations"=w2826, "Injection Times"=w2828, "Enable Start Retry"=w2824, "Day/Night Cycle"=w2829, "Final Start Presses"=w2817, "Semaphore"=w2819) -> ("GUI Aisle 1"=w2837:T3[], "Test Station Out"=w2832:T7, "Enable Start Retry Out"=w2825:bool[], "Error Out"=w2834:errorcluster)  [unwired: 5 in, 1 out]
        n1445 = call <vilib>:"Add State(s) to Queue__jki_lib_state_machine.vi"("State(s) in (\"\")"=w2842) -> ("States Out"=w2841:string)  [unwired: 14 in]
        n1446 = Bundle By Name(cluster=w2840, "GUI Aisle 1 (SLAT)."=w2837, "Station Test State Cluster"=w2832, "Enable Start Retry Array"=w2825) -> (w2839:T24)
      }
      frame "Station 4" {
        w2860 = 3  # Aisle Location Index
        w2863 = u32 4  # Station Number
        # "Control the state of station 4"
        n1447 = Unbundle By Name(w2867) -> ("Enable Start Retry Array"=w2852:bool[], "Agilent Switches"=w2853:T2[], "GUI Aisle 1 (SLAT)."=w2865:T3[], "Drying Time (Min)"=w2848:dbl[], "Current Threshold"=w2854:dbl, "Station Test State Cluster"=w2858:T7, "Station Timeout Values (1-56) Seconds"=w2849:dbl[], "Send Restart Every? (Sec)"=w2850:dbl, "Injection Times Input"=w2855:T15, "Day/Night Cycle Input"=w2856:T11)
        n1448 = local read "Delay After Cutout (Sec)"() -> (w2845:dbl)
        n1449 = local read "Final Start Presses"() -> (w2844:i32)
        n1450 = local read "Agilent Semaphore"() -> (w2846:T1[])
        n1451 = local read "Previous Run Statistics"() -> (w2847:T9[])
        n1452 = local read "Disable Flood Check"() -> (w2843:bool)
        n1453 = call "WILT Station Controller.vi"("Station Number"=w2863, "GUI Aisle in"=w2865, "Drying Time (Min)"=w2848, "Current Threshold"=w2854, "Station Test State In"=w2858, "Error In"=w2862, "Aisle Location Index"=w2860, "Cool Down Period (seconds)"=w2849, "Disable Flood Check"=w2843, "Delay After Cutout (sec)"=w2845, "Previous Run Statistics"=w2847, "Send Restart Every? (Sec)"=w2850, "Agilent Valve and Switch Locations"=w2853, "Injection Times"=w2855, "Enable Start Retry"=w2852, "Day/Night Cycle"=w2856, "Final Start Presses"=w2844, "Semaphore"=w2846) -> ("GUI Aisle 1"=w2864:T3[], "Test Station Out"=w2859:T7, "Enable Start Retry Out"=w2851:bool[], "Error Out"=w2861:errorcluster)  [unwired: 5 in, 1 out]
        n1454 = Bundle By Name(cluster=w2867, "GUI Aisle 1 (SLAT)."=w2864, "Station Test State Cluster"=w2859, "Enable Start Retry Array"=w2851) -> (w2866:T24)
        n1455 = call <vilib>:"Add State(s) to Queue__jki_lib_state_machine.vi"("State(s) in (\"\")"=w2869) -> ("States Out"=w2868:string)  [unwired: 14 in]
      }
      frame "Station 5" {
        w2887 = 4  # Aisle Location Index
        w2890 = u32 5  # Station Number
        # "Control the state of station 5"
        n1456 = Unbundle By Name(w2894) -> ("Enable Start Retry Array"=w2879:bool[], "Agilent Switches"=w2881:T2[], "GUI Aisle 1 (SLAT)."=w2892:T3[], "Drying Time (Min)"=w2875:dbl[], "Current Threshold"=w2880:dbl, "Station Test State Cluster"=w2885:T7, "Station Timeout Values (1-56) Seconds"=w2876:dbl[], "Send Restart Every? (Sec)"=w2877:dbl, "Injection Times Input"=w2882:T15, "Day/Night Cycle Input"=w2883:T11)
        n1457 = local read "Delay After Cutout (Sec)"() -> (w2872:dbl)
        n1458 = local read "Final Start Presses"() -> (w2871:i32)
        n1459 = local read "Agilent Semaphore"() -> (w2873:T1[])
        n1460 = local read "Previous Run Statistics"() -> (w2874:T9[])
        n1461 = local read "Disable Flood Check"() -> (w2870:bool)
        n1462 = call "WILT Station Controller.vi"("Station Number"=w2890, "GUI Aisle in"=w2892, "Drying Time (Min)"=w2875, "Current Threshold"=w2880, "Station Test State In"=w2885, "Error In"=w2889, "Aisle Location Index"=w2887, "Cool Down Period (seconds)"=w2876, "Disable Flood Check"=w2870, "Delay After Cutout (sec)"=w2872, "Previous Run Statistics"=w2874, "Send Restart Every? (Sec)"=w2877, "Agilent Valve and Switch Locations"=w2881, "Injection Times"=w2882, "Enable Start Retry"=w2879, "Day/Night Cycle"=w2883, "Final Start Presses"=w2871, "Semaphore"=w2873) -> ("GUI Aisle 1"=w2891:T3[], "Test Station Out"=w2886:T7, "Enable Start Retry Out"=w2878:bool[], "Error Out"=w2888:errorcluster)  [unwired: 5 in, 1 out]
        n1463 = call <vilib>:"Add State(s) to Queue__jki_lib_state_machine.vi"("State(s) in (\"\")"=w2896) -> ("States Out"=w2895:string)  [unwired: 14 in]
        n1464 = Bundle By Name(cluster=w2894, "GUI Aisle 1 (SLAT)."=w2891, "Station Test State Cluster"=w2886, "Enable Start Retry Array"=w2878) -> (w2893:T24)
      }
      frame "Station 6" {
        w2914 = 5  # Aisle Location Index
        w2917 = u32 6  # Station Number
        # "Control the state of station 6"
        n1465 = Unbundle By Name(w2921) -> ("Enable Start Retry Array"=w2906:bool[], "Agilent Switches"=w2908:T2[], "GUI Aisle 1 (SLAT)."=w2919:T3[], "Drying Time (Min)"=w2902:dbl[], "Current Threshold"=w2907:dbl, "Station Test State Cluster"=w2912:T7, "Station Timeout Values (1-56) Seconds"=w2903:dbl[], "Send Restart Every? (Sec)"=w2904:dbl, "Injection Times Input"=w2909:T15, "Day/Night Cycle Input"=w2910:T11)
        n1466 = local read "Delay After Cutout (Sec)"() -> (w2899:dbl)
        n1467 = local read "Final Start Presses"() -> (w2898:i32)
        n1468 = local read "Agilent Semaphore"() -> (w2900:T1[])
        n1469 = local read "Previous Run Statistics"() -> (w2901:T9[])
        n1470 = local read "Disable Flood Check"() -> (w2897:bool)
        n1471 = call "WILT Station Controller.vi"("Station Number"=w2917, "GUI Aisle in"=w2919, "Drying Time (Min)"=w2902, "Current Threshold"=w2907, "Station Test State In"=w2912, "Error In"=w2916, "Aisle Location Index"=w2914, "Cool Down Period (seconds)"=w2903, "Disable Flood Check"=w2897, "Delay After Cutout (sec)"=w2899, "Previous Run Statistics"=w2901, "Send Restart Every? (Sec)"=w2904, "Agilent Valve and Switch Locations"=w2908, "Injection Times"=w2909, "Enable Start Retry"=w2906, "Day/Night Cycle"=w2910, "Final Start Presses"=w2898, "Semaphore"=w2900) -> ("GUI Aisle 1"=w2918:T3[], "Test Station Out"=w2913:T7, "Enable Start Retry Out"=w2905:bool[], "Error Out"=w2915:errorcluster)  [unwired: 5 in, 1 out]
        n1472 = Bundle By Name(cluster=w2921, "GUI Aisle 1 (SLAT)."=w2918, "Station Test State Cluster"=w2913, "Enable Start Retry Array"=w2905) -> (w2920:T24)
        n1473 = call <vilib>:"Add State(s) to Queue__jki_lib_state_machine.vi"("State(s) in (\"\")"=w2923) -> ("States Out"=w2922:string)  [unwired: 14 in]
      }
      frame "Station 7" {
        w2941 = 6  # Aisle Location Index
        w2944 = u32 7  # Station Number
        # "Control the state of station 7"
        n1474 = Unbundle By Name(w2948) -> ("Enable Start Retry Array"=w2932:bool[], "Agilent Switches"=w2935:T2[], "GUI Aisle 1 (SLAT)."=w2946:T3[], "Drying Time (Min)"=w2929:dbl[], "Current Threshold"=w2934:dbl, "Station Test State Cluster"=w2939:T7, "Station Timeout Values (1-56) Seconds"=w2930:dbl[], "Send Restart Every? (Sec)"=w2931:dbl, "Injection Times Input"=w2936:T15, "Day/Night Cycle Input"=w2937:T11)
        n1475 = local read "Delay After Cutout (Sec)"() -> (w2926:dbl)
        n1476 = local read "Final Start Presses"() -> (w2925:i32)
        n1477 = local read "Agilent Semaphore"() -> (w2927:T1[])
        n1478 = local read "Previous Run Statistics"() -> (w2928:T9[])
        n1479 = local read "Disable Flood Check"() -> (w2924:bool)
        n1480 = call "WILT Station Controller.vi"("Station Number"=w2944, "GUI Aisle in"=w2946, "Drying Time (Min)"=w2929, "Current Threshold"=w2934, "Station Test State In"=w2939, "Error In"=w2943, "Aisle Location Index"=w2941, "Cool Down Period (seconds)"=w2930, "Disable Flood Check"=w2924, "Delay After Cutout (sec)"=w2926, "Previous Run Statistics"=w2928, "Send Restart Every? (Sec)"=w2931, "Agilent Valve and Switch Locations"=w2935, "Injection Times"=w2936, "Enable Start Retry"=w2932, "Day/Night Cycle"=w2937, "Final Start Presses"=w2925, "Semaphore"=w2927) -> ("GUI Aisle 1"=w2945:T3[], "Test Station Out"=w2940:T7, "Enable Start Retry Out"=w2933:bool[], "Error Out"=w2942:errorcluster)  [unwired: 5 in, 1 out]
        n1481 = Bundle By Name(cluster=w2948, "GUI Aisle 1 (SLAT)."=w2945, "Station Test State Cluster"=w2940, "Enable Start Retry Array"=w2933) -> (w2947:T24)
        n1482 = call <vilib>:"Add State(s) to Queue__jki_lib_state_machine.vi"("State(s) in (\"\")"=w2950) -> ("States Out"=w2949:string)  [unwired: 14 in]
      }
      frame "Station 8" {
        w2968 = 7  # Aisle Location Index
        w2971 = u32 8  # Station Number
        # "Control the state of station 8"
        n1483 = Unbundle By Name(w2975) -> ("Enable Start Retry Array"=w2959:bool[], "Agilent Switches"=w2962:T2[], "GUI Aisle 1 (SLAT)."=w2973:T3[], "Drying Time (Min)"=w2956:dbl[], "Current Threshold"=w2961:dbl, "Station Test State Cluster"=w2966:T7, "Station Timeout Values (1-56) Seconds"=w2957:dbl[], "Send Restart Every? (Sec)"=w2958:dbl, "Injection Times Input"=w2963:T15, "Day/Night Cycle Input"=w2964:T11)
        n1484 = local read "Delay After Cutout (Sec)"() -> (w2953:dbl)
        n1485 = local read "Final Start Presses"() -> (w2952:i32)
        n1486 = local read "Agilent Semaphore"() -> (w2954:T1[])
        n1487 = local read "Previous Run Statistics"() -> (w2955:T9[])
        n1488 = local read "Disable Flood Check"() -> (w2951:bool)
        n1489 = call "WILT Station Controller.vi"("Station Number"=w2971, "GUI Aisle in"=w2973, "Drying Time (Min)"=w2956, "Current Threshold"=w2961, "Station Test State In"=w2966, "Error In"=w2970, "Aisle Location Index"=w2968, "Cool Down Period (seconds)"=w2957, "Disable Flood Check"=w2951, "Delay After Cutout (sec)"=w2953, "Previous Run Statistics"=w2955, "Send Restart Every? (Sec)"=w2958, "Agilent Valve and Switch Locations"=w2962, "Injection Times"=w2963, "Enable Start Retry"=w2959, "Day/Night Cycle"=w2964, "Final Start Presses"=w2952, "Semaphore"=w2954) -> ("GUI Aisle 1"=w2972:T3[], "Test Station Out"=w2967:T7, "Enable Start Retry Out"=w2960:bool[], "Error Out"=w2969:errorcluster)  [unwired: 5 in, 1 out]
        n1490 = Bundle By Name(cluster=w2975, "GUI Aisle 1 (SLAT)."=w2972, "Station Test State Cluster"=w2967, "Enable Start Retry Array"=w2960) -> (w2974:T24)
        n1491 = call <vilib>:"Add State(s) to Queue__jki_lib_state_machine.vi"("State(s) in (\"\")"=w2977) -> ("States Out"=w2976:string)  [unwired: 14 in]
      }
      frame "Station 9" {
        w2995 = 8  # Aisle Location Index
        w2998 = u32 9  # Station Number
        # "Control the state of station 9"
        n1492 = Unbundle By Name(w3002) -> ("Enable Start Retry Array"=w2987:bool[], "Agilent Switches"=w2988:T2[], "GUI Aisle 1 (SLAT)."=w3000:T3[], "Drying Time (Min)"=w2982:dbl[], "Current Threshold"=w2989:dbl, "Station Test State Cluster"=w2993:T7, "Station Timeout Values (1-56) Seconds"=w2984:dbl[], "Send Restart Every? (Sec)"=w2985:dbl, "Injection Times Input"=w2990:T15, "Day/Night Cycle Input"=w2991:T11)
        n1493 = local read "Previous Run Statistics"() -> (w2983:T9[])
        n1494 = local read "Disable Flood Check"() -> (w2978:bool)
        n1495 = local read "Delay After Cutout (Sec)"() -> (w2980:dbl)
        n1496 = local read "Final Start Presses"() -> (w2979:i32)
        n1497 = local read "Agilent Semaphore"() -> (w2981:T1[])
        n1498 = call "WILT Station Controller.vi"("Station Number"=w2998, "GUI Aisle in"=w3000, "Drying Time (Min)"=w2982, "Current Threshold"=w2989, "Station Test State In"=w2993, "Error In"=w2997, "Aisle Location Index"=w2995, "Cool Down Period (seconds)"=w2984, "Disable Flood Check"=w2978, "Delay After Cutout (sec)"=w2980, "Previous Run Statistics"=w2983, "Send Restart Every? (Sec)"=w2985, "Agilent Valve and Switch Locations"=w2988, "Injection Times"=w2990, "Enable Start Retry"=w2987, "Day/Night Cycle"=w2991, "Final Start Presses"=w2979, "Semaphore"=w2981) -> ("GUI Aisle 1"=w2999:T3[], "Test Station Out"=w2994:T7, "Enable Start Retry Out"=w2986:bool[], "Error Out"=w2996:errorcluster)  [unwired: 5 in, 1 out]
        n1499 = Bundle By Name(cluster=w3002, "GUI Aisle 1 (SLAT)."=w2999, "Station Test State Cluster"=w2994, "Enable Start Retry Array"=w2986) -> (w3001:T24)
        n1500 = call <vilib>:"Add State(s) to Queue__jki_lib_state_machine.vi"("State(s) in (\"\")"=w3004) -> ("States Out"=w3003:string)  [unwired: 14 in]
      }
      frame "Station 10" {
        w3022 = 9  # Aisle Location Index
        w3025 = u32 10  # Station Number
        # "Control the state of station 10"
        n1501 = Unbundle By Name(w3029) -> ("Enable Start Retry Array"=w3014:bool[], "Agilent Switches"=w3016:T2[], "GUI Aisle 1 (SLAT)."=w3027:T3[], "Drying Time (Min)"=w3010:dbl[], "Current Threshold"=w3015:dbl, "Station Test State Cluster"=w3020:T7, "Station Timeout Values (1-56) Seconds"=w3011:dbl[], "Send Restart Every? (Sec)"=w3012:dbl, "Injection Times Input"=w3017:T15, "Day/Night Cycle Input"=w3018:T11)
        n1502 = local read "Previous Run Statistics"() -> (w3009:T9[])
        n1503 = local read "Disable Flood Check"() -> (w3005:bool)
        n1504 = local read "Delay After Cutout (Sec)"() -> (w3007:dbl)
        n1505 = local read "Final Start Presses"() -> (w3006:i32)
        n1506 = local read "Agilent Semaphore"() -> (w3008:T1[])
        n1507 = call "WILT Station Controller.vi"("Station Number"=w3025, "GUI Aisle in"=w3027, "Drying Time (Min)"=w3010, "Current Threshold"=w3015, "Station Test State In"=w3020, "Error In"=w3024, "Aisle Location Index"=w3022, "Cool Down Period (seconds)"=w3011, "Disable Flood Check"=w3005, "Delay After Cutout (sec)"=w3007, "Previous Run Statistics"=w3009, "Send Restart Every? (Sec)"=w3012, "Agilent Valve and Switch Locations"=w3016, "Injection Times"=w3017, "Enable Start Retry"=w3014, "Day/Night Cycle"=w3018, "Final Start Presses"=w3006, "Semaphore"=w3008) -> ("GUI Aisle 1"=w3026:T3[], "Test Station Out"=w3021:T7, "Enable Start Retry Out"=w3013:bool[], "Error Out"=w3023:errorcluster)  [unwired: 5 in, 1 out]
        n1508 = Bundle By Name(cluster=w3029, "GUI Aisle 1 (SLAT)."=w3026, "Station Test State Cluster"=w3021, "Enable Start Retry Array"=w3013) -> (w3028:T24)
        n1509 = call <vilib>:"Add State(s) to Queue__jki_lib_state_machine.vi"("State(s) in (\"\")"=w3031) -> ("States Out"=w3030:string)  [unwired: 14 in]
      }
      frame "Station 11" {
        w3049 = 10  # Aisle Location Index
        w3052 = u32 11  # Station Number
        # "Control the state of station 11"
        n1510 = Unbundle By Name(w3056) -> ("Enable Start Retry Array"=w3041:bool[], "Agilent Switches"=w3043:T2[], "GUI Aisle 1 (SLAT)."=w3054:T3[], "Drying Time (Min)"=w3037:dbl[], "Current Threshold"=w3042:dbl, "Station Test State Cluster"=w3047:T7, "Station Timeout Values (1-56) Seconds"=w3038:dbl[], "Send Restart Every? (Sec)"=w3039:dbl, "Injection Times Input"=w3044:T15, "Day/Night Cycle Input"=w3045:T11)
        n1511 = local read "Previous Run Statistics"() -> (w3036:T9[])
        n1512 = local read "Disable Flood Check"() -> (w3032:bool)
        n1513 = local read "Delay After Cutout (Sec)"() -> (w3034:dbl)
        n1514 = local read "Final Start Presses"() -> (w3033:i32)
        n1515 = local read "Agilent Semaphore"() -> (w3035:T1[])
